vi "CreateProfileToSave.vi"(11 "Input Array":dbl[](array[numeric])) -> (2 "Ouput array":dbl[](array[numeric]))   [LabVIEW 2022 SP3]
panel:
  out "size(s)":i32
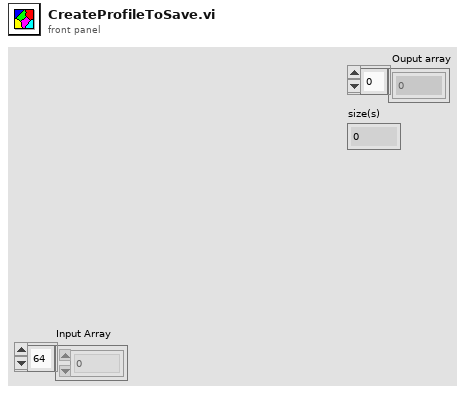
[diagram p1: front panel]
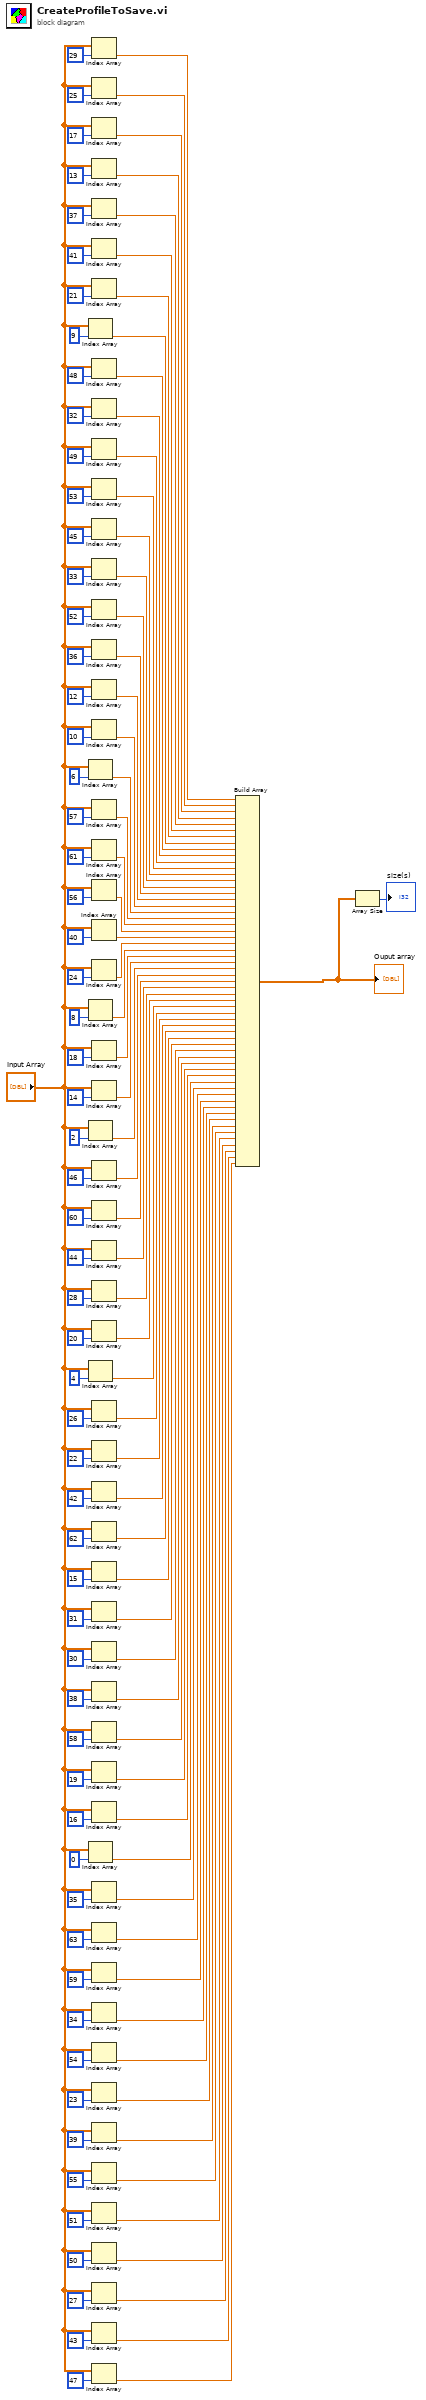
[diagram p0: block diagram]
diagram:
  n1 = Index Array(array="Input Array", index=9) -> (element=w55:dbl)
  n2 = Index Array(array="Input Array", index=6) -> (element=w44:dbl)
  n3 = Index Array(array="Input Array", index=8) -> (element=w38:dbl)
  n4 = Index Array(array="Input Array", index=2) -> (element=w35:dbl)
  n5 = Index Array(array="Input Array", index=4) -> (element=w28:dbl)
  n6 = Index Array(array="Input Array", index=0) -> (element=w16:dbl)
  n7 = Index Array(array="Input Array", index=29) -> (element=w62:dbl)
  n8 = Index Array(array="Input Array", index=25) -> (element=w61:dbl)
  n9 = Index Array(array="Input Array", index=17) -> (element=w60:dbl)
  n10 = Index Array(array="Input Array", index=13) -> (element=w59:dbl)
  n11 = Index Array(array="Input Array", index=37) -> (element=w58:dbl)
  n12 = Index Array(array="Input Array", index=41) -> (element=w57:dbl)
  n13 = Index Array(array="Input Array", index=21) -> (element=w56:dbl)
  n14 = Index Array(array="Input Array", index=48) -> (element=w54:dbl)
  n15 = Index Array(array="Input Array", index=32) -> (element=w53:dbl)
  n16 = Index Array(array="Input Array", index=49) -> (element=w52:dbl)
  n17 = Index Array(array="Input Array", index=53) -> (element=w51:dbl)
  n18 = Index Array(array="Input Array", index=45) -> (element=w50:dbl)
  n19 = Index Array(array="Input Array", index=33) -> (element=w49:dbl)
  n20 = Index Array(array="Input Array", index=52) -> (element=w48:dbl)
  n21 = Index Array(array="Input Array", index=36) -> (element=w47:dbl)
  n22 = Index Array(array="Input Array", index=12) -> (element=w46:dbl)
  n23 = Index Array(array="Input Array", index=10) -> (element=w45:dbl)
  n24 = Index Array(array="Input Array", index=57) -> (element=w43:dbl)
  n25 = Index Array(array="Input Array", index=61) -> (element=w42:dbl)
  n26 = Index Array(array="Input Array", index=56) -> (element=w41:dbl)
  n27 = Index Array(array="Input Array", index=40) -> (element=w40:dbl)
  n28 = Index Array(array="Input Array", index=24) -> (element=w39:dbl)
  n29 = Index Array(array="Input Array", index=18) -> (element=w37:dbl)
  n30 = Index Array(array="Input Array", index=14) -> (element=w36:dbl)
  n31 = Index Array(array="Input Array", index=46) -> (element=w34:dbl)
  n32 = Index Array(array="Input Array", index=60) -> (element=w33:dbl)
  n33 = Index Array(array="Input Array", index=44) -> (element=w32:dbl)
  n34 = Index Array(array="Input Array", index=28) -> (element=w31:dbl)
  n35 = Index Array(array="Input Array", index=20) -> (element=w30:dbl)
  n36 = Index Array(array="Input Array", index=26) -> (element=w27:dbl)
  n37 = Index Array(array="Input Array", index=22) -> (element=w26:dbl)
  n38 = Index Array(array="Input Array", index=42) -> (element=w25:dbl)
  n39 = Index Array(array="Input Array", index=62) -> (element=w24:dbl)
  n40 = Index Array(array="Input Array", index=15) -> (element=w23:dbl)
  n41 = Index Array(array="Input Array", index=31) -> (element=w22:dbl)
  n42 = Index Array(array="Input Array", index=30) -> (element=w21:dbl)
  n43 = Index Array(array="Input Array", index=38) -> (element=w20:dbl)
  n44 = Index Array(array="Input Array", index=58) -> (element=w19:dbl)
  n45 = Index Array(array="Input Array", index=19) -> (element=w18:dbl)
  n46 = Index Array(array="Input Array", index=16) -> (element=w17:dbl)
  n47 = Index Array(array="Input Array", index=35) -> (element=w15:dbl)
  n48 = Index Array(array="Input Array", index=63) -> (element=w14:dbl)
  n49 = Index Array(array="Input Array", index=59) -> (element=w13:dbl)
  n50 = Index Array(array="Input Array", index=34) -> (element=w12:dbl)
  n51 = Index Array(array="Input Array", index=54) -> (element=w11:dbl)
  n52 = Index Array(array="Input Array", index=23) -> (element=w10:dbl)
  n53 = Index Array(array="Input Array", index=39) -> (element=w9:dbl)
  n54 = Index Array(array="Input Array", index=55) -> (element=w8:dbl)
  n55 = Index Array(array="Input Array", index=51) -> (element=w7:dbl)
  n56 = Index Array(array="Input Array", index=50) -> (element=w6:dbl)
  n57 = Index Array(array="Input Array", index=27) -> (element=w5:dbl)
  n58 = Index Array(array="Input Array", index=43) -> (element=w4:dbl)
  n59 = Index Array(array="Input Array", index=47) -> (element=w3:dbl)
  n60 = Build Array(w62, w61, w60, w59, w58, w57, w56, w55, w54, w53, w52, w51, w50, w49, w48, w47, w46, w45, w44, w43, w42, w41, w40, w39, w38, w37, w36, w35, w34, w33, w32, w31, w30, w28, w27, w26, w25, w24, w23, w22, w21, w20, w19, w18, w17, w16, w15, w14, w13, w12, w11, w10, w9, w8, w7, w6, w5, w4, w3) -> (w2:dbl[])
  "Ouput array" <- w2
  n61 = Array Size(array=w2) -> (size(s)=→"size(s)":i32)
